vi "1 Channel 1 Sample - Manual Timestamp.vi"() -> ()   [LabVIEW 2026, in "synnax_clib.lvlib"]
uses:
  lvlib/synnax_clib.lvlib
  lvlib/typedefs/connection_config.ctl
  lvlib/classes/Client/Private/synnax channel retrieve keys Single.vi
  lvlib/classes/Writer/Private/synnax writer open Array.vi
  lvlib/classes/Writer/Private/Writes/DBL/Write 1Ch 1Samp (DBL).vi
  lvlib/classes/Synnax Writer.lvclass
  lvlib/classes/Client/Synnax Client.lvclass
panel:
  in  "Channel":string="my_f64_chan"
  out "cos(x)":dbl
  in  "Stop":bool
  out "error out":errorcluster
  in  "Connection Config":T1={"host"="localhost", "port"=9090, "username"="synnax", "password"="seldon"}
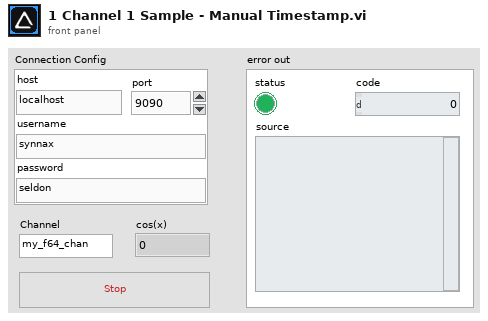
[diagram p1: front panel]
types:
  T1 = typedef "synnax_clib.lvlib/connection_config.ctl" = cluster{"host":string, "port":u16, "username":string, "password":string}
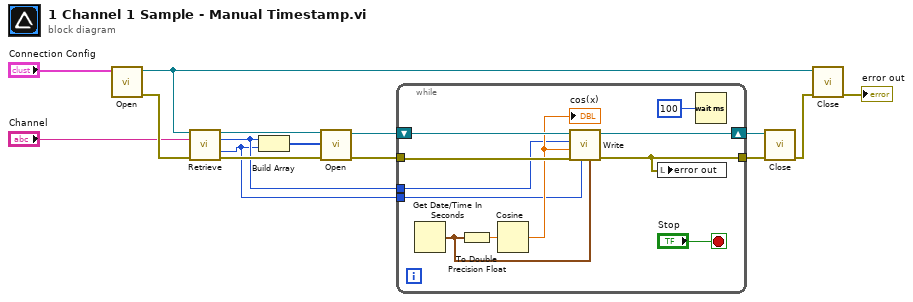
[diagram p0: block diagram]
diagram:
  n1 = call "Open.vi"("Connection Config"="Connection Config") -> ("error out"=w10:errorcluster, "Synnax Client out"=w12:refnum<class "Synnax Client.lvclass">)  [unwired: 9 in]
  n2 = call-poly "Retrieve.vi"("Synnax Client in"=w12, "channel name"="Channel", "error in"=w10) -> ("Synnax Client out"=w6:refnum<class "Synnax Client.lvclass">, "channel key"=w2:u32, "index key"=w1:u32, "error out"=w14:errorcluster)  [unwired: 8 in, 1 out]
  n3 = Build Array(w2, w1) -> (w3:u32[])
  n4 = call-poly "Open.vi"("error in"=w14, "channels in"=w3, "Synnax Client in"=w6) -> ("error out"=w7:errorcluster, "writer out"=w9:refnum<class "Synnax Writer.lvclass">)  [unwired: 6 in, 1 out]
  n5 = while {
    shift-right: [w25] -> w8
    shift-left: w9 -> [w26]
    tunnel: w7 -> [w24]
    tunnel: [w20] -> w15
    tunnel: w1 -> [w18]
    tunnel: w2 -> [w16]
    stop <- "Stop" stop-if-true
    n6 = Get Date/Time In Seconds() -> (seconds since 1Jan1904=w17:timestamp)
    n7 = To Double Precision Float(number=w17) -> (double precision float=w19:dbl)
    n8 = Cosine(x=w19) -> (cos(x)=w22:dbl)
    "cos(x)" <- w22
    n9 = call-poly "Write.vi"("timestamp"=w17, "index_channel"=w18, "error in"=w24, "data"=w22, "channel"=w16, "Writer"=w26) -> ("error out"=w20:errorcluster, "Writer Out"=w25:refnum<class "Synnax Writer.lvclass">)  [unwired: 4 in]
    n10 = local write "error out"(w20) -> ()
    n11 = Wait (ms)(milliseconds to wait=u32 100) -> ()  [unwired: 1 out]
  }
  n12 = call "Close.vi"("error in"=w15, "writer"=w8) -> ("error out"=w11:errorcluster)  [unwired: 9 in]
  n13 = call "Close.vi"("error in"=w11, "Synnax Client in"=w12) -> ("error out"=→"error out":errorcluster)  [unwired: 9 in]
